vi "Template.vi"(8 "Error In":errorcluster, 11 "App cluster in":T1={"s"}) -> (0 "Error Out":errorcluster, 3 "App cluster Out":T1={"s"})   [LabVIEW 2024]
uses:
  Controls/App Cluster.ctl
panel:
  # "Inputs to the VI"
  # "Outputs from the VI"
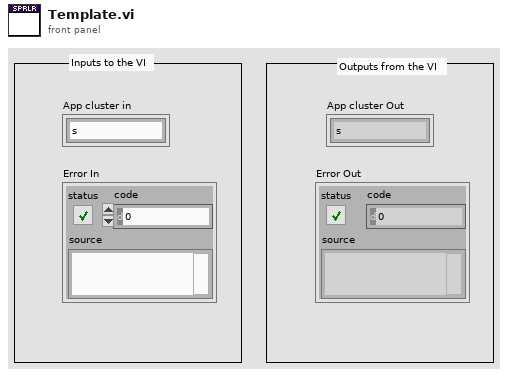
[diagram p1: front panel]
types:
  T1 = typedef "App Cluster.ctl" = cluster{string}
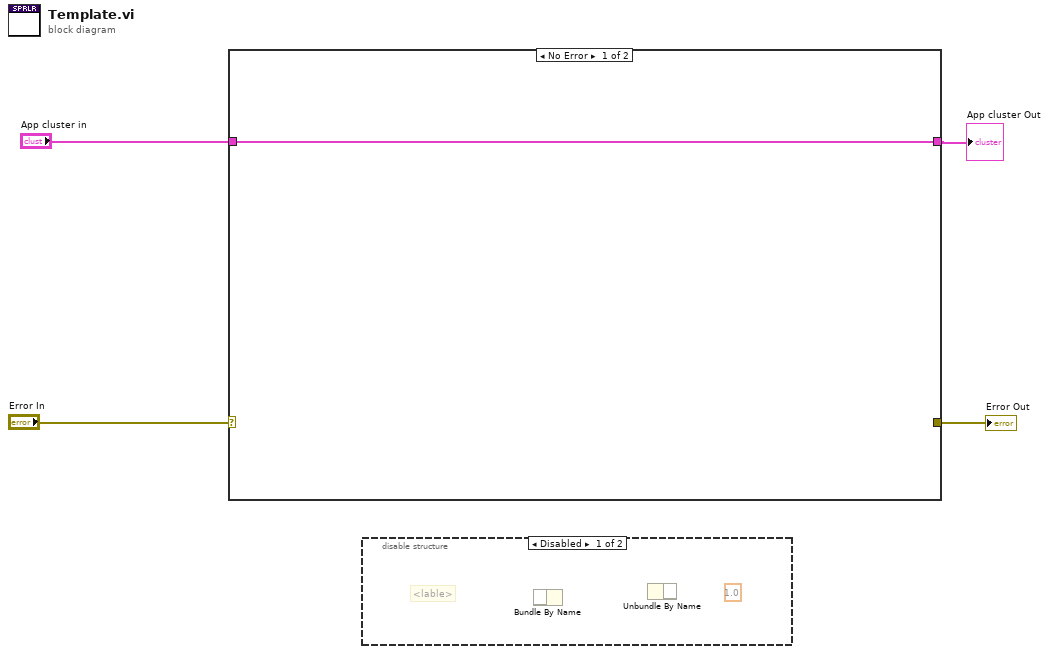
[diagram p0: block diagram]
diagram:
  n1 = case shown="No Error" "Error In" {
    selector: "Error In" -> [_ w6]
    tunnel: [_ w6] -> w4
    tunnel: "App cluster in" -> [w5 _]
    tunnel: [w5 _] -> w1
    frame No Error {
    }
    frame Error {
      # "Pass through the error"
    }
  }
  "Error Out" <- w4
  "App cluster Out" <- w1
  n2 = disable-structure shown="Disabled" {
    frame Disabled {
      (unwired) 1.0
      # "<lable>"
      n3 = Bundle By Name() -> ()  [unwired: 2 in, 1 out]
      n4 = Unbundle By Name() -> ()  [unwired: 1 in, 1 out]
    }
    frame Enabled {
    }
  }
